vi "Stop VIs Stream.vi"(8 "error in (no error)":errorcluster, 11 "Channel in":refnum<class "Channel.lvclass">) -> (0 "error out":errorcluster, 3 "Channel out":refnum<class "Channel.lvclass">)   [LabVIEW 2018, in "Channel.lvclass"]
doc: "Stop the VI responsible for communication"
uses:
  Channel.lvclass
  Channel.lvclass/Channel.ctl
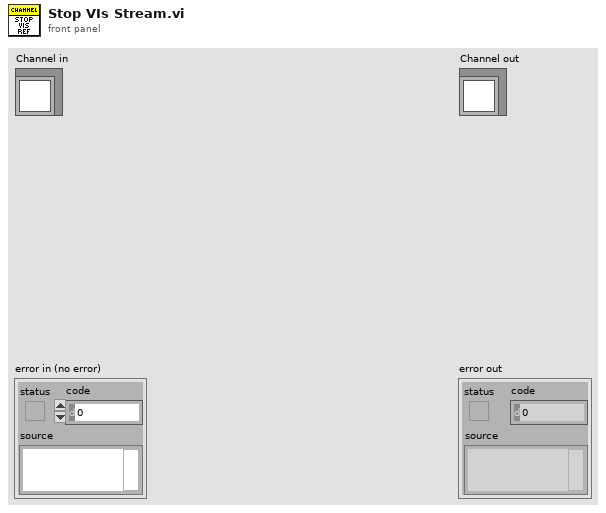
[diagram p1: front panel]
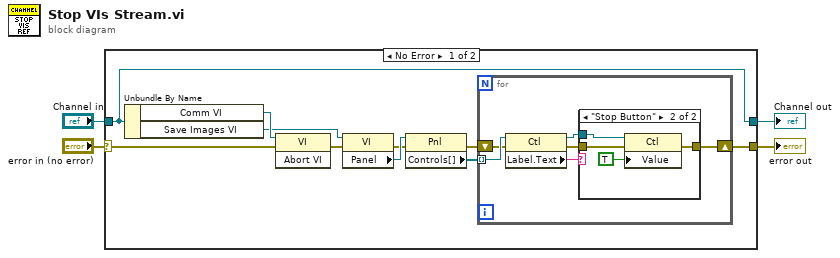
[diagram p0: block diagram]
diagram:
  n1 = case shown="No Error" "error in (no error)" {
    selector: "error in (no error)" -> [w11 w27]
    tunnel: [w13 w27] -> w3
    tunnel: [w14 w26] -> w1
    tunnel: "Channel in" -> [w14 w26]
    frame No Error {
      n2 = Unbundle By Name(w14) -> ("Comm VI"=w12:refnum<vi>, "Save Images VI"=w5:refnum<vi>)
      n3 = invoke class="VI" method="Abort VI"(reference=w12, error in=w11) -> (error out=w10:errorcluster)  [unwired: 1 in, 2 out]
      n4 = property class="VI"(reference=w5, error in=w10) -> (error out=w7:errorcluster, "Panel"=w9:refnum<vi>)  [unwired: 1 out]
      n5 = property class="Pnl"(reference=w9, error in=w7) -> (error out=w6:errorcluster, "Controls[]"=w8:refnum<vi>[])  [unwired: 1 out]
      n6 = for {
        tunnel: w8 -> [w20] mode=indexing
        shift-right: [w15] -> w13
        shift-left: w6 -> [w17]
        n7 = property class="Ctl"(reference=w20, error in=w17) -> (reference out=w18:refnum<vi>, error out=w16:errorcluster, "Label.Text"=w19:string)
        n8 = case shown="\"Stop Button\"" w19 {
          tunnel: w18 -> [_ w25]
          tunnel: w16 -> [w21 w23]
          tunnel: [w21 w22] -> w15
          frame "False", Default {
          }
          frame "Stop Button" {
            n9 = property class="Ctl"(reference=w25, error in=w23, "Value"=TRUE) -> (error out=w22:errorcluster)  [unwired: 1 out]
          }
        }
      }
    }
    frame Error {
    }
  }
  "error out" <- w3
  "Channel out" <- w1
